vi "Obtain References.vi"(7 "Path to Project":path, 8 "error in (no error)":errorcluster) -> (0 "error out":errorcluster, 3 "References":T1, 5 "FPGA Target Found":bool)   [LabVIEW 2014, in "SPI Engine Scripting.lvlib"]
uses:
  SPI Engine Scripting.lvlib
  Supporting VIs/References.ctl
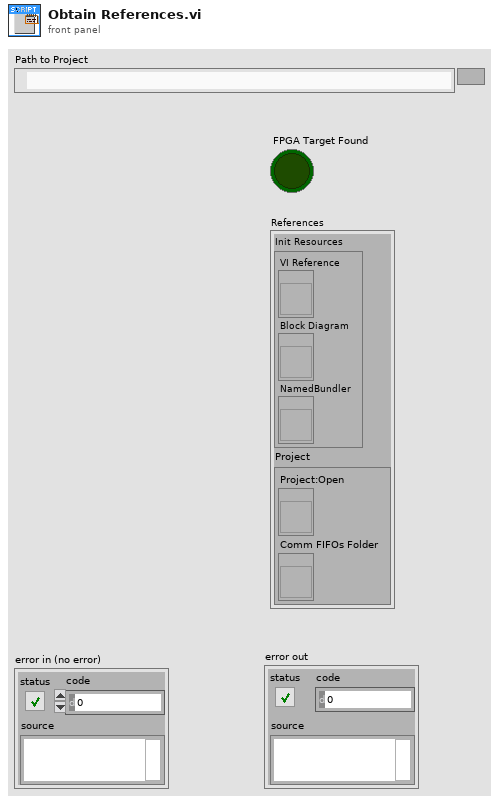
[diagram p1: front panel]
types:
  T1 = typedef "SPI Engine Scripting.lvlib/References.ctl" = cluster{"Init Resources":cluster{"VI Reference":refnum<vi>, "Block Diagram":refnum<vi>, "NamedBundler":refnum<vi>}, "Project":cluster{"Project:Open":refnum<vi>, "Comm FIFOs Folder":refnum<vi>}}
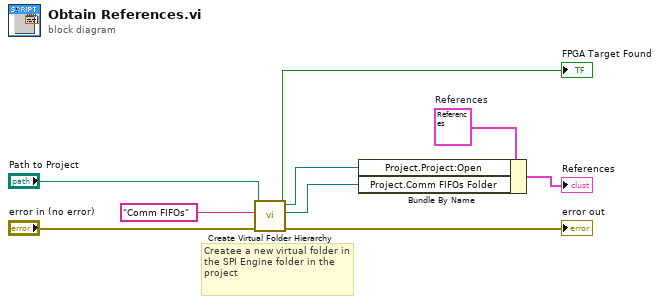
[diagram p0: block diagram]
diagram:
  w8 = T1 {"Init Resources"={"VI Reference"=refnum, "Block Diagram"=refnum, "NamedBundler"=refnum}, "Project"={"Project:Open"=refnum, "Comm FIFOs Folder"=refnum}}  # References
  # "Createe a new virtual folder in the SPI Engine folder in the project"
  n1 = call "Create Virtual Folder Hierarchy.vi"("error in"="error in (no error)", "Virtual Folder Name"="Comm FIFOs", "Path to Project"="Path to Project") -> ("error out"=→"error out":errorcluster, "FPGA Target Found"=→"FPGA Target Found":bool, "New Virtual Folder"=w4:refnum<vi>, "Project:Open"=w3:refnum<vi>)  [unwired: 5 in]
  n2 = Bundle By Name(cluster=w8, "Project.Project:Open"=w3, "Project.Comm FIFOs Folder"=w4) -> (→"References":T1)
